vi "Main.vi"() -> ()   [LabVIEW 2016]
panel:
  in  "Stop_button":bool
  in  "Door_position":bool
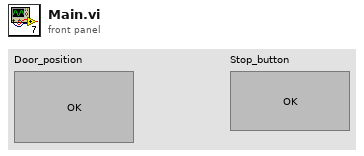
[diagram p1: front panel]
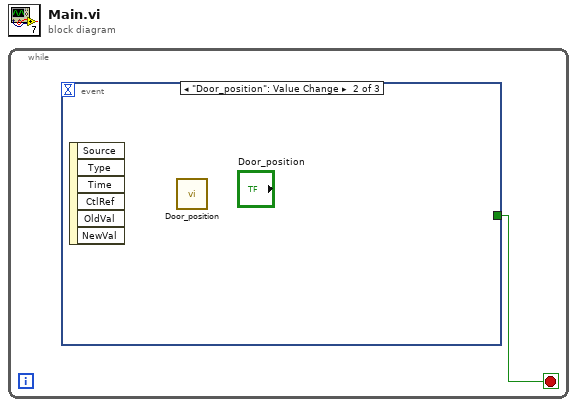
[diagram p0: block diagram]
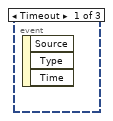
[diagram p2: hidden frame]
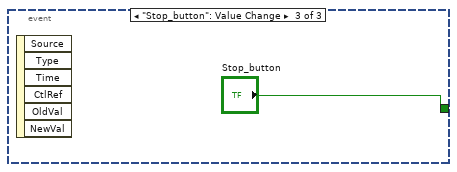
[diagram p3: hidden frame]
diagram:
  n1 = while {
    stop <- w1 stop-if-true
    n2 = event shown="[1] \"Door_position\": Value Change" {
      selector: _ -> [_ _ _]
      dyn-events: _ -> [_ _ _]
      timeout: _ -> [_ _ _]
      tunnel: [_ _ "Stop_button"] -> w1
      event Timeout {
        n3 = event-data() -> ()  [unwired: 1 in, 3 out]
      }
      event "Door_position": Value Change {
        n4 = event-data() -> ()  [unwired: 1 in, 6 out]
        n5 = call "Door_position.vi"() -> ()  [unwired: 12 in]
      }
      event "Stop_button": Value Change {
        n6 = event-data() -> ()  [unwired: 1 in, 6 out]
      }
    }
  }
